vi "SetTimeout.vi"(8 "error in (no error)":errorcluster, 10 "value in":dbl, 11 "Photometrics Cam v2 in":refnum<class "Photometrics_CH-250_Cam.lvclass">) -> (0 "error out":errorcluster, 2 "value out":dbl, 3 "Photometrics Cam v2 out":refnum<class "Photometrics_CH-250_Cam.lvclass">)   [LabVIEW 2013, in "Photometrics_CH-250_Cam.lvclass"]
uses:
  Photometrics_CH-250_Cam.lvclass
  Photometrics_CH-250_Cam.lvclass/Photometrics_CH-250_Cam.ctl
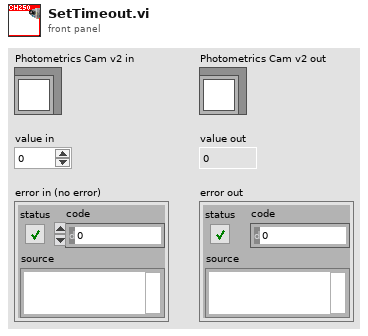
[diagram p1: front panel]
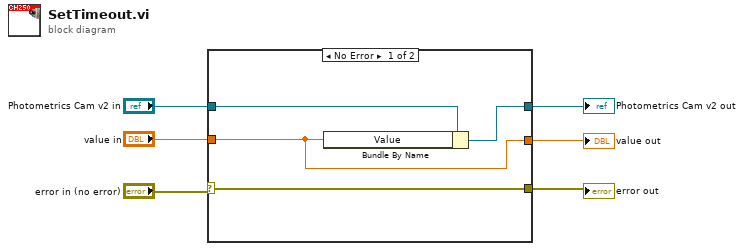
[diagram p0: block diagram]
diagram:
  n1 = case shown="No Error" "error in (no error)" {
    selector: "error in (no error)" -> [w8 w13]
    tunnel: "Photometrics Cam v2 in" -> [w10 w12]
    tunnel: [w9 w12] -> w2
    tunnel: "value in" -> [w7 w11]
    tunnel: [w8 w13] -> w4
    tunnel: [w7 w11] -> w6
    frame No Error {
      n2 = Bundle By Name(cluster=w10, "Value"=w7) -> (w9:refnum<class "Photometrics_CH-250_Cam.lvclass">)
    }
    frame Error {
    }
  }
  "value out" <- w6
  "error out" <- w4
  "Photometrics Cam v2 out" <- w2
